vi "3a_lit_num.vi"(4 "erreur in":errorcluster caption="err in", 6 "varid":T1, 7 "tdms file in":refnum<k34>) -> (0 "error out":errorcluster caption="err out", 1 "do_num":T5, 2 "varid":T1, 3 "tdms file out":refnum<k34>)   [LabVIEW 2010, in "lv_04.lvlib"]
uses:
  lv_04.lvlib
  commandes/cSTA_varid.ctl
  commandes/c_TDMS_ch_variable.ctl
  commandes/c_TDMS_ch_donnees.ctl
  commandes/c0-var-n.ctl
  commandes/c02-do-num.ctl
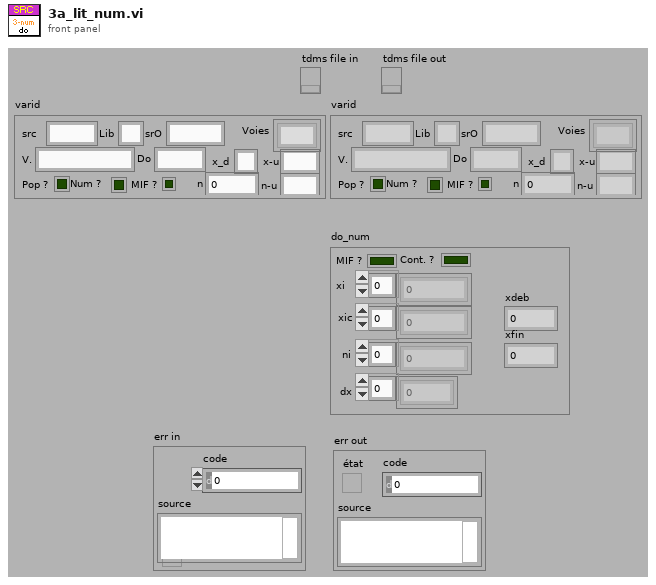
[diagram p1: front panel]
types:
  T1 = typedef "lv_04.lvlib/cSTA_varid.ctl" = cluster{"src":string, "Lib":string, "srO":string, "V.":T2, "Voies":string[], "Do":T3, "n":T4, "Num ?":bool, "Pop ?":bool, "x_d":string, "x-u":string, "n-u":string, "MIF ?":bool}
  T2 = typedef "lv_04.lvlib/c_TDMS_ch_variable.ctl" = string
  T3 = typedef "lv_04.lvlib/c_TDMS_ch_donnees.ctl" = string
  T4 = typedef "lv_04.lvlib/c0-var-n.ctl" = i32
  T5 = typedef "lv_04.lvlib/c02-do-num.ctl" = cluster{"MIF ?":bool, "Cont. ?":bool, "xi":dbl[], "xic":dbl[], "ni":u32[], "dx":dbl[], "xdeb":dbl, "xfin":dbl}
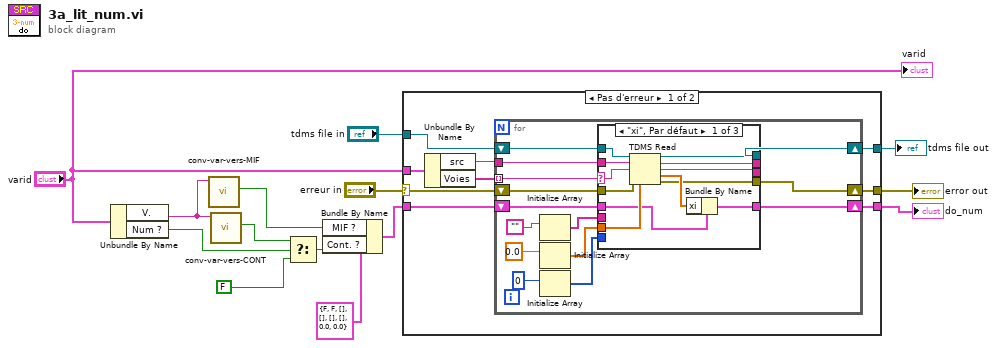
[diagram p0: block diagram]
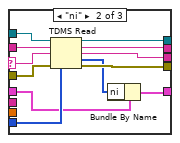
[diagram p2: hidden frame]
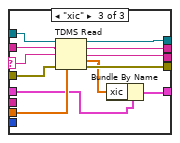
[diagram p3: hidden frame]
diagram:
  n1 = Unbundle By Name("varid") -> ("V."=w4:T2, "Num ?"=w6:bool)
  n2 = call "conv-var-vers-MIF.vi"("Variable"=w4) -> ("MIF ?"=w7:bool)  [unwired: 4 in, 2 out]
  n3 = call "conv-var-vers-CONT.vi"("Variable"=w4) -> ("Cont. ?"=w2:bool)  [unwired: 4 in, 2 out]
  n4 = Select(t=w2, s=w6, f=FALSE) -> (s? t:f=w1:bool)
  n5 = Bundle By Name(cluster=T5 {"MIF ?"=FALSE, "Cont. ?"=FALSE, "xi"=[], "xic"=[], "ni"=[], "dx"=[], "xdeb"=0.0, "xfin"=0.0} ("X_num 2"), "MIF ?"=w7, "Cont. ?"=w1) -> (w8:T5)
  n6 = case shown="Pas d'erreur" "erreur in" {
    selector: "erreur in" -> [w23 w74]
    tunnel: "tdms file in" -> [w15 w76]
    tunnel: [w22 w76] -> w12
    tunnel: "varid" -> [w21 _]
    tunnel: [w20 w75] -> w11
    tunnel: w8 -> [w19 w75]
    tunnel: [w16 w74] -> w10
    frame No Error {
      n7 = Unbundle By Name(w21) -> ("src"=w17:string, "Voies"=w18:string[])
      n8 = for {
        tunnel: w18 -> [w37] mode=indexing
        tunnel: w17 -> [w33]
        shift-right: [w31] -> w16
        shift-left: w23 -> [w30]
        shift-right: [w25] -> w20
        shift-left: w19 -> [w26]
        shift-right: [w24] -> w22
        shift-left: w15 -> [w32]
        n9 = Initialize Array("") -> (w35:string[])  [unwired: 1 in]
        n10 = Initialize Array(0.0) -> (w34:dbl[])  [unwired: 1 in]
        n11 = Initialize Array(0) -> (w27:i32[])  [unwired: 1 in]
        n12 = case shown="\"xi\", Par défaut" w37 {
          selector: w37 -> [w47 w61 w68]
          tunnel: w35 -> [_ _ _]
          tunnel: w34 -> [w45 _ w73]
          tunnel: w33 -> [w48 w59 w67]
          tunnel: w32 -> [w49 w60 w66]
          tunnel: [w38 w53 w70] -> w31
          tunnel: w30 -> [w46 w58 w69]
          tunnel: [w41 w56 w65] -> w24
          tunnel: w27 -> [_ w57 _]
          tunnel: w26 -> [w44 w54 w71]
          tunnel: [w42 w55 w72] -> w25
          tunnel: [w40 w51 w63] -> _
          tunnel: [w39 w50 w62] -> _
          frame "xi", Default {
            n13 = TDMS Read(0:w49, 5:w48, 7:w47, 11:w46, 12:w45) -> (4:w41:refnum<k34>, 6:w40:string, 8:w39:string, 10:w43:dbl[], 15:w38:errorcluster)  [unwired: 2 in, 1 out]
            n14 = Bundle By Name(cluster=w44, "xi"=w43) -> (w42:T5)
          }
          frame "ni" {
            n15 = TDMS Read(0:w60, 5:w59, 7:w61, 11:w58, 12:w57) -> (4:w56:refnum<k34>, 6:w51:string, 8:w50:string, 10:w52:i32[], 15:w53:errorcluster)  [unwired: 2 in, 1 out]
            n16 = Bundle By Name(cluster=w54, "ni"=w52) -> (w55:T5)
          }
          frame "xic" {
            n17 = TDMS Read(0:w66, 5:w67, 7:w68, 11:w69, 12:w73) -> (4:w65:refnum<k34>, 6:w63:string, 8:w62:string, 10:w64:dbl[], 15:w70:errorcluster)  [unwired: 2 in, 1 out]
            n18 = Bundle By Name(cluster=w71, "xic"=w64) -> (w72:T5)
          }
        }
      }
    }
    frame Error {
    }
  }
  "error out" <- w10
  "tdms file out" <- w12
  "do_num" <- w11
  "varid" <- "varid"
